vi "Unit_vector_gen.vi"(11 "Length":i32) -> (3 "Unit_length_Vector":dbl[](array[numeric]))   [LabVIEW 2014]
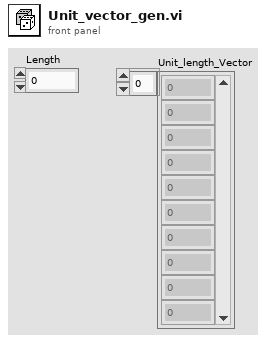
[diagram p1: front panel]
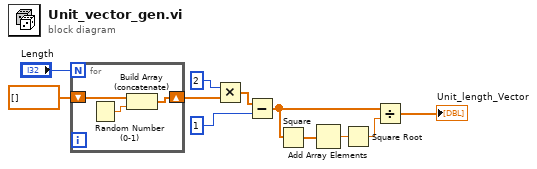
[diagram p0: block diagram]
diagram:
  n1 = for {
    N: "Length" -> [_]
    shift-right: [w13] -> w9
    shift-left: dbl[] [] -> [w12]
    n2 = Random Number (0-1)() -> (number: 0 to 1=w14:dbl)
    n3 = Build Array (concatenate)(w12, w14) -> (w13:dbl[])
  }
  n4 = Multiply(x=2, y=w9) -> (x*y=w7:dbl[])
  n5 = Subtract(x=w7, y=1) -> (x-y=w2:dbl[])
  n6 = Square(x=w2) -> (x^2=w5:dbl[])
  n7 = Add Array Elements(numeric array=w5) -> (sum=w4:dbl)
  n8 = Square Root(x=w4) -> (sqrt(x)=w3:dbl)
  n9 = Divide(x=w2, y=w3) -> (x/y=→"Unit_length_Vector":dbl[])
